vi "Initialize.vi"(7 "Option String":string, 8 "error in (no error)":errorcluster, 9 "btnReset":bool caption="Reset (F)", 10 "btnIdQuery":bool caption="Id Query (F)", 11 "NhRegenGridSim in":refnum<class "NhRegenGridSim.lvclass">) -> (0 "error out":errorcluster, 3 "NhRegenGridSim out":refnum<class "NhRegenGridSim.lvclass">)   [LabVIEW 2018, in "AcPwrPlugins.lvlib" / "NhRegenGridSim.lvclass"]
doc: "This VI opens a connection to all phases. It optionally resets the phase or checks that the phase ID is valid."
uses:
  NhRegenGridSim.lvclass
  NhRegenGridSim.lvclass/NhRegenGridSim.ctl
  Accessors/Read Loads.vi
  Accessors/Write Loads.vi
  <instrlib>/NH Research 9400 Series/NH Research 9400 Series.lvlib
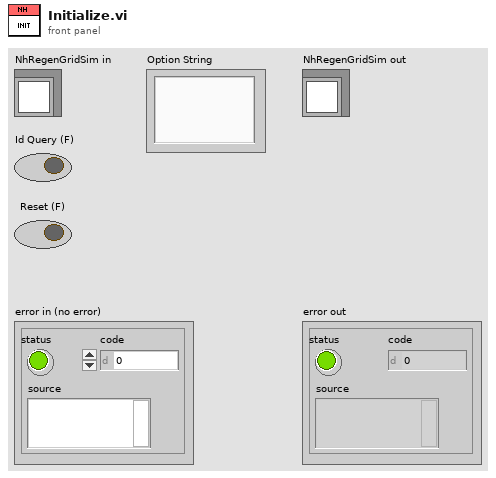
[diagram p1: front panel]
types:
  T1 = typedef "AcPwrPlugins.lvlib/NhRegenGridSim.lvclass/Load.ctl" = cluster{"SlewRates":cluster{"Islew":dbl, "Vslew":dbl, "Pslew":dbl, "FreqSlew":dbl, "AngleABSlew":dbl, "AngleACSlew":dbl}, "Phases":cluster{"Pout":dbl, "Iout":dbl, "PhaseAngle":dbl, "Vout":dbl, "Phase Name":string}[], "Measurement":cluster{"ApertureLength":dbl, "NumberOfSamples":u32}, "Ranges":cluster{"Irange":dbl, "Vrange":dbl}, "Mode":enum8{"One 3-Phase AC", "One AC", "One DC", "Three AC", "Three DC", "One 2-Phase AC and One AC", "One 2-Phase AC and One DC", "Two AC", "One AC and One DC", "Two AC and One DC", "One AC and Two DC", "One DC and One AC", "Two DC"}, "PowerMax":u16, "TransformerRatio":dbl, "Waveshape":dbl[], "Handle":string, "FreqOut":dbl, "Connected":bool, "Safety Limits":cluster{"Minimum Voltage (V)":dbl, "Minimum Voltage Time (s)":dbl, "Maximum Voltage (V)":dbl, "Maximum Voltage Time (s)":dbl, "Maximum Source Amps (A)":dbl, "Maximum Source Amps Time (s)":dbl, "Maximum Sink Amps (A)":dbl, "Maximum Sink Amps Time (s)":dbl, "Maximum Source Power (W)":dbl, "Maximum Source Power Time (s)":dbl, "Maximum Sink Power (W)":dbl, "Maximum Sink Power Time (s)":dbl, "Peak Voltage (V)":dbl, "Peak Voltage Enable":bool, "Peak Amps (A)":dbl, "Peak Amps Enable":bool}}
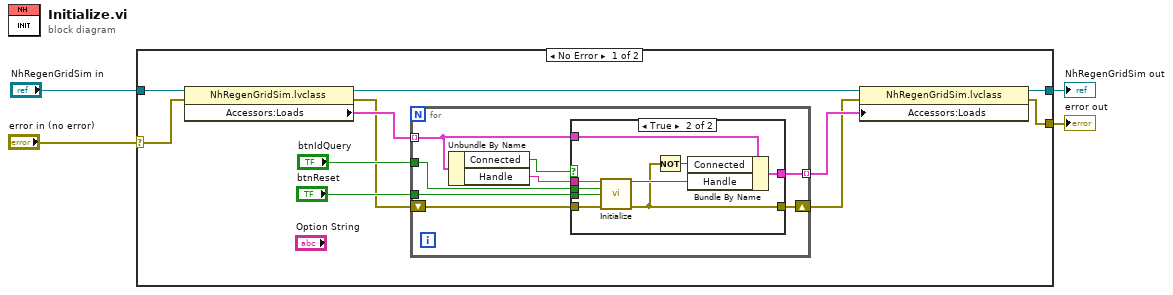
[diagram p0: block diagram]
diagram:
  n1 = case shown="No Error" "error in (no error)" {
    selector: "error in (no error)" -> [w9 w35]
    tunnel: "NhRegenGridSim in" -> [w13 w36]
    tunnel: [w6 w36] -> w2
    tunnel: [w5 w35] -> w1
    frame No Error {
      n2 = property class="NhRegenGridSim.lvclass"(reference=w13, error in=w9) -> (reference out=w10:refnum<class "NhRegenGridSim.lvclass">, error out=w8:errorcluster, "Accessors:Loads"=w12:T1[])
      n3 = for {
        shift-right: [w22] -> w7
        shift-left: w8 -> [w23]
        tunnel: "btnReset" -> [w21]
        tunnel: "btnIdQuery" -> [w20]
        tunnel: w12 -> [w18] mode=indexing
        tunnel: [w17] -> w11 mode=indexing
        n4 = Unbundle By Name(w18) -> ("Connected"=w16:bool, "Handle"=w19:string)
        n5 = case shown="True" w16 {
          tunnel: w23 -> [w25 w34]
          tunnel: [w25 w26] -> w22
          tunnel: w21 -> [_ w33]
          tunnel: w20 -> [_ w32]
          tunnel: w19 -> [_ w31]
          tunnel: w18 -> [w24 w30]
          tunnel: [w24 w28] -> w17
          frame False {
          }
          frame True {
            n6 = call <instrlib>:"Initialize.vi"("VISA resource name"=w31, "ID Query (True)"=w32, "Reset (True)"=w33, "error in (no error)"=w34) -> ("VISA resource name out"=w29:refnum<visa-resource-name>, "error out"=w26:errorcluster)  [unwired: 10 in]
            n7 = Not(x=w26) -> (.not. x?=w27:bool)
            n8 = Bundle By Name(cluster=w30, "Connected"=w27, "Handle"=w29) -> (w28:T1)
          }
        }
      }
      n9 = property class="NhRegenGridSim.lvclass"(reference=w10, error in=w7, "Accessors:Loads"=w11) -> (reference out=w6:refnum<class "NhRegenGridSim.lvclass">, error out=w5:errorcluster)
    }
    frame Error {
    }
  }
  "error out" <- w1
  "NhRegenGridSim out" <- w2
